vi "Clean Up Message Handler.vi"(6 "Acknowledge Data in":T1, 8 "error in":errorcluster, 11 "Response String":string) -> (0 "error out":errorcluster, 4 "Acknowledge Data out":T1)   [LabVIEW 2015, in "Generic Module Library.lvlib" / "Template G_Module.lvlib"]
uses:
  Template G_Module.lvlib
  Private Controls/Module Message Cluster Components/Acknowledge Data Cluster.ctl
  Private Controls/Module Message Cluster Components/Ack Payload.ctl
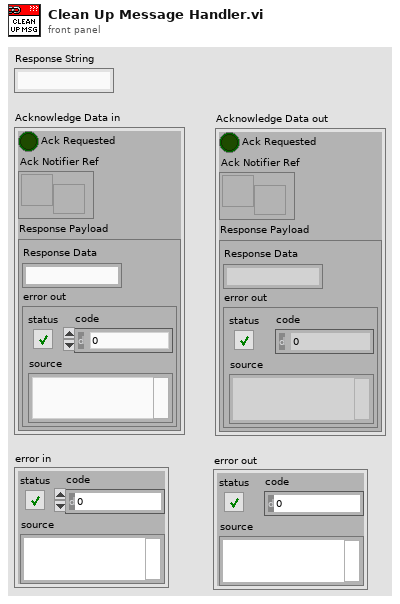
[diagram p1: front panel]
types:
  T1 = typedef "Generic Module Library.lvlib/Template G_Module.lvlib/Acknowledge Data Cluster.ctl" = cluster{"Ack Requested":bool, "Ack Notifier Ref":refnum<notifier>, "Response Payload":T2}
  T2 = typedef "Generic Module Library.lvlib/Template G_Module.lvlib/Ack Payload.ctl" = cluster{"Response Data":string, "error out":errorcluster}
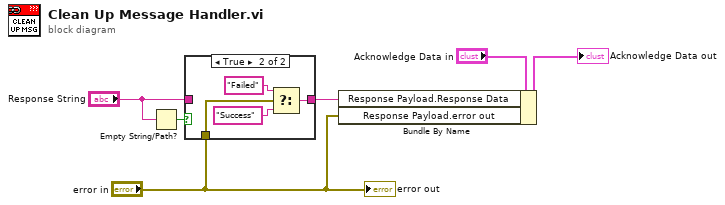
[diagram p0: block diagram]
diagram:
  n1 = Empty String/Path?(string/path="Response String") -> (empty?=w3:bool)
  n2 = case shown="True" w3 {
    tunnel: [w7 w8] -> w5
    tunnel: "Response String" -> [w7 _]
    tunnel: "error in" -> [_ w9]
    frame False {
    }
    frame True {
      n3 = Select(t="Failed", s=w9, f="Success") -> (s? t:f=w8:string)
    }
  }
  n4 = Bundle By Name(cluster="Acknowledge Data in", "Response Payload.Response Data"=w5, "Response Payload.error out"="error in") -> (→"Acknowledge Data out":T1)
  "error out" <- "error in"
